vi "LowLvCtrl_Init.vi"(7 "Encoder Tasks In":tag[](array[tag]), 8 "error in (no error)":errorcluster, 9 "Analog Task In":refnum<k21>="LoadCells_FSR_AI", 10 "FPGA VI Reference In":refnum<k20>) -> (0 "error out":errorcluster, 3 "LowLvControl":T1)   [LabVIEW 2016]
uses:
  TypeDef/LowLvControl Cluster.ctl
  Classes/MotorControl/MotorControl.lvclass
  <vilib>/DAQmx/create/channels.llb/DAQmx Create Channel (CI-Position-Angular Encoder).vi
  <vilib>/FPGAPlugInAG/Dynamic/niLvFpga_Run_Dynamic.vi
  <vilib>/FPGAPlugInAG/Dynamic/niLvFpga_Reset_Dynamic.vi
  <vilib>/Utility/error.llb/Error Cluster From Error Code.vi
  <vilib>/rvi/errors/niLvFpgaAdjustHostInterfaceError.vi
  <vilib>/rvi/interface/nirviMethod/nirviMethod.xnode
  <vilib>/rvi/interface/nirviReadWriteControl/nirviReadWriteControl.xnode
  NiFpgaLv.dll
  <vilib>/rvi/interface/Simulation/niFpgaSimulationCallBeginRW.vi
panel:
  in  "MTP Files":cluster{"Motor ID":i32, "Tuning File":path}[](array[cluster])=[{"Motor ID"=4, "Tuning File"=path "c:/MotorParam/eci40-4-1.mtp"}, {"Motor ID"=5, "Tuning File"=path "c:/MotorParam/eci40-5-1.mtp"}, {"Motor ID"=6, "Tuning File"=path "c:/MotorParam/eci40-6-1.mtp"}, {"Motor ID"=7, "Tuning File"=path "c:/MotorParam/eci40-7-1.mtp"}]
  in  "decoding type":i32(ring)=10092 items=["X1"=10090, "X2"=10091, "X4"=10092, "Two Pulse Counting"=10313]
  in  "units":i32(ring)=10273 items=["Degrees"=10146, "Radians"=10273, "Ticks"=10304, "From Custom Scale"=10065]
  in  "CPR":u32=2048
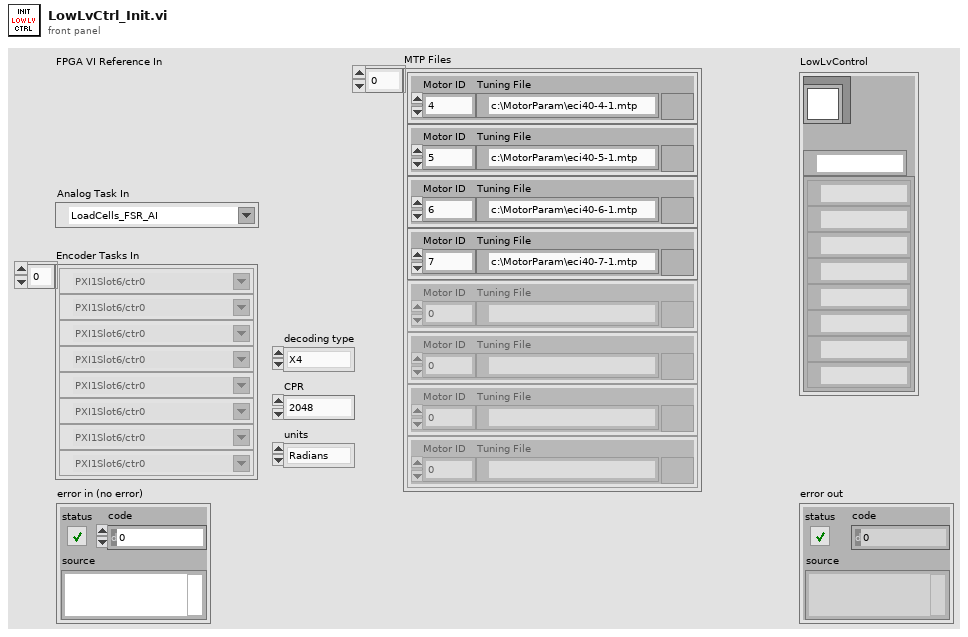
[diagram p1: front panel]
types:
  T1 = typedef "LowLvControl Cluster.ctl" = cluster{"MotorCtrl":refnum<class "MotorControl.lvclass">, "FPGA Ref":refnum<k20>, "AI Task":refnum<k21>, "Encoder Tasks":refnum<k21>[]}
  T2 = cluster{"Input":enum16{"Fr:Cable", "Fr:Motor", "Fr:Sensor"}, "Output":enum16{"To:Cable", "To:Motor", "To:Sensor"}}
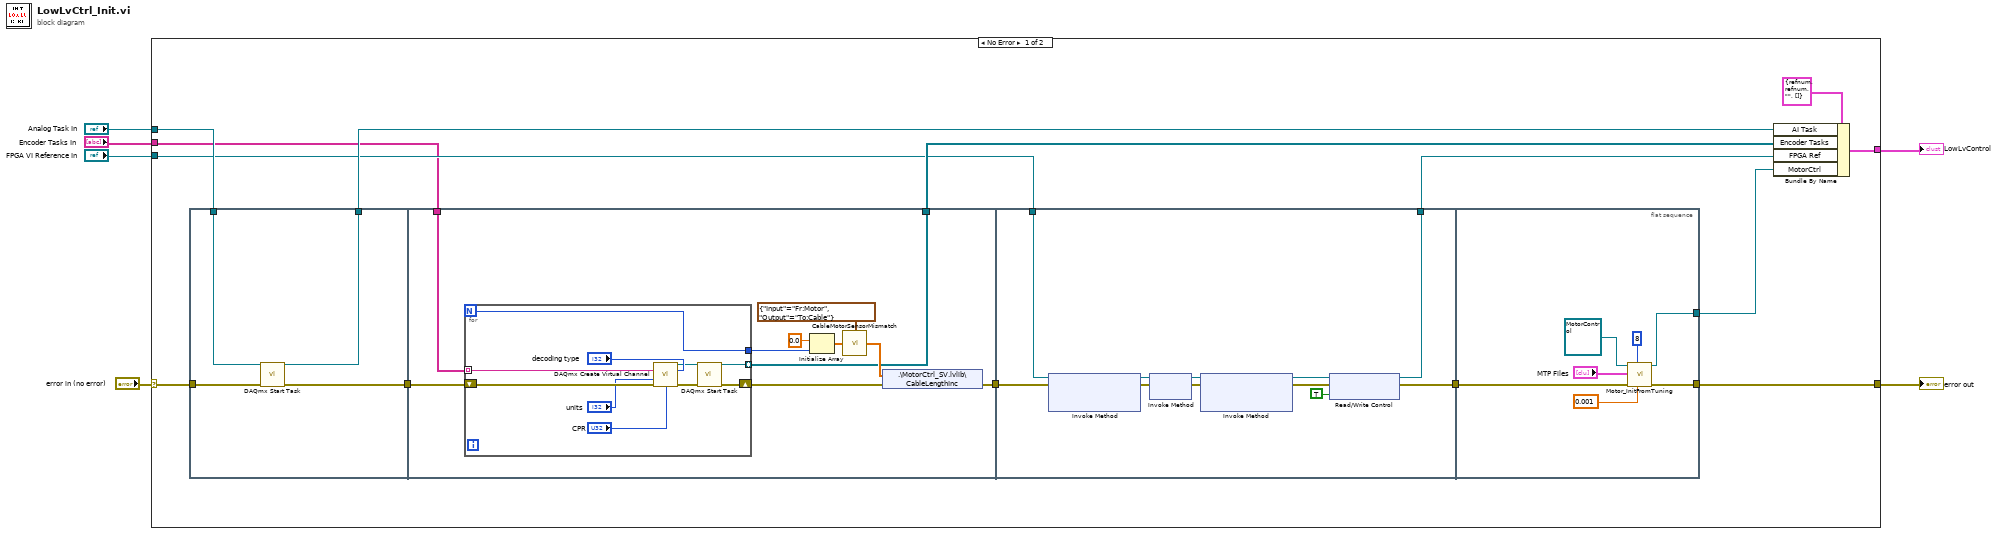
[diagram p0: block diagram]
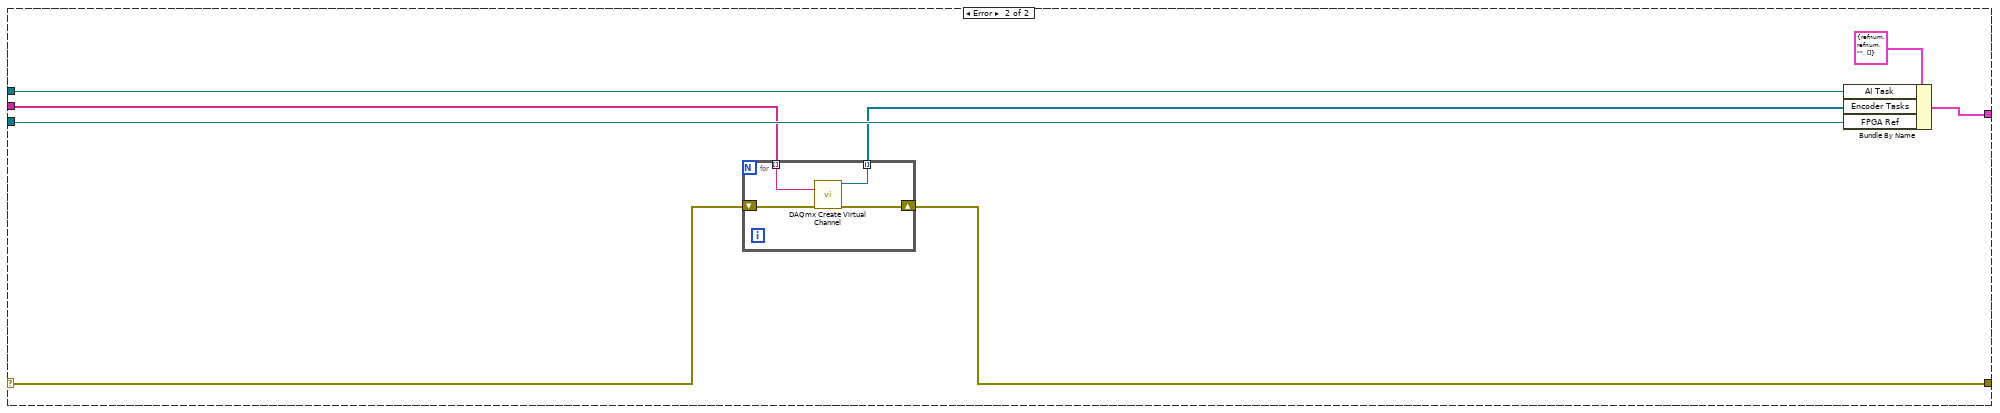
[diagram p2: hidden frame]
diagram:
  n1 = case shown="No Error" "error in (no error)" {
    selector: "error in (no error)" -> [w10 w64]
    tunnel: [w17 w63] -> w6
    tunnel: [w14 w69] -> w5
    tunnel: "Analog Task In" -> [w9 w68]
    tunnel: "FPGA VI Reference In" -> [w8 w67]
    tunnel: "Encoder Tasks In" -> [w7 w66]
    frame No Error {
      n2 = flat-sequence {
        tunnel: w10 -> [w24]
        tunnel: [w23] -> w20
        tunnel: [w22] -> w11
        tunnel: w9 -> [w21]
        tunnel: w20 -> [w28]
        tunnel: [w27] -> w19
        tunnel: [w26] -> w12
        tunnel: w7 -> [w25]
        tunnel: w19 -> [w51]
        tunnel: [w48] -> w18
        tunnel: [w46] -> w13
        tunnel: w8 -> [w45]
        tunnel: w18 -> [w62]
        tunnel: [w61] -> w17
        tunnel: [w60] -> w15
        frame #0 {
          n3 = call <vilib>:"DAQmx Start Task.vi"("task/channels in"=w21, "error in"=w24) -> ("task out"=w22:refnum<k21>, "error out"=w23:errorcluster)  [unwired: 12 in]
        }
        frame #1 {
          n4 = for {
            N -> [w35]
            tunnel: w25 -> [w44] mode=indexing
            tunnel: [w38] -> w26 mode=indexing
            shift-right: [w36] -> w31
            shift-left: w28 -> [w41]
            tunnel: [w35] -> w29
            n5 = call-poly <vilib>:"DAQmx Create Virtual Channel.vi"("counter"=w44, "decoding type"="decoding type", "units"="units", "error in"=w41, "pulses per revolution"="CPR") -> ("task out"=w39:refnum<k21>, "error out"=w37:errorcluster)  [unwired: 9 in]
            n6 = call <vilib>:"DAQmx Start Task.vi"("task/channels in"=w39, "error in"=w37) -> ("task out"=w38:refnum<k21>, "error out"=w36:errorcluster)  [unwired: 12 in]
          }
          n7 = Initialize Array(0.0, w29) -> (w32:dbl[])
          n8 = call "CableMotorSensorMismatch.vi"("Conversion"=T2 {"Input"=enum."Fr:Motor", "Output"=enum."To:Cable"}, "Input"=w32) -> ("Output"=w33:dbl[])  [unwired: 2 in]
          n9 = shared-variable ".\\MotorCtrl_SV.lvlib\\CableLengthInc"(w33, error in=w31) -> (error out=w27:errorcluster)
        }
        frame #2 {
          n10 = xnode "Invoke Method"("FPGA VI Reference In"=w45, "error in"=w51) -> ("FPGA VI Reference Out"=w52:refnum<k20>, "error out"=w53:errorcluster)  [unwired: 1 in]
          n11 = xnode "Invoke Method"("FPGA VI Reference In"=w52, "error in"=w53) -> ("FPGA VI Reference Out"=w54:refnum<k20>, "error out"=w55:errorcluster)
          n12 = xnode "Invoke Method"("FPGA VI Reference In"=w54, "error in"=w55) -> ("FPGA VI Reference Out"=w50:refnum<k20>, "error out"=w49:errorcluster)  [unwired: 1 in]
          n13 = xnode "Read/Write Control"("FPGA VI Reference In"=w50, "error in"=w49, "EnableMaster"=TRUE) -> ("FPGA VI Reference Out"=w46:refnum<k20>, "error out"=w48:errorcluster)
        }
        frame #3 {
          n14 = call "Motor_InitFromTuning.vi"("PID LoopPeriod(s)"=0.001, "Motor Quantity (0: Use Tuning Files Quantity)"=8, "error in (no error)"=w62, "Motor Tuning Files"="MTP Files", "MotorCtrl in"=refnum<class "MotorControl.lvclass"> refnum ("MotorCtrl")) -> ("error out"=w61:errorcluster, "MotorCtrl out"=w60:refnum<class "MotorControl.lvclass">)  [unwired: 5 in]
        }
      }
      n15 = Bundle By Name(cluster=T1 {"MotorCtrl"=refnum, "FPGA Ref"=refnum, "AI Task"="", "Encoder Tasks"=[]} ("LowLvControl"), "AI Task"=w11, "Encoder Tasks"=w12, "FPGA Ref"=w13, "MotorCtrl"=w15) -> (w14:T1)
    }
    frame Error {
      n16 = for {
        tunnel: w66 -> [w74] mode=indexing
        tunnel: [w73] -> w65 mode=indexing
        shift-right: [w71] -> w63
        shift-left: w64 -> [w72]
        n17 = call-poly <vilib>:"DAQmx Create Virtual Channel.vi"("counter"=w74, "error in"=w72) -> ("task out"=w73:refnum<k21>, "error out"=w71:errorcluster)  [unwired: 12 in]
      }
      n18 = Bundle By Name(cluster=T1 {"MotorCtrl"=refnum, "FPGA Ref"=refnum, "AI Task"="", "Encoder Tasks"=[]} ("LowLvControl"), "AI Task"=w68, "Encoder Tasks"=w65, "FPGA Ref"=w67) -> (w69:T1)
    }
  }
  "error out" <- w6
  "LowLvControl" <- w5
